vi "Mood Analysis.vi"(2 "Rhythm":dbl[][](array[numeric]), 3 "Timbre":dbl[][](array[numeric]), 4 "Intensity":dbl[][](array[numeric])) -> (0 "Stress":dbl, 1 "Energy":dbl)   [LabVIEW 2013]
panel:
  out "Mood Group":i16(graph)
  out "Stress":dbl(graph)
  out "Energy":dbl(graph)
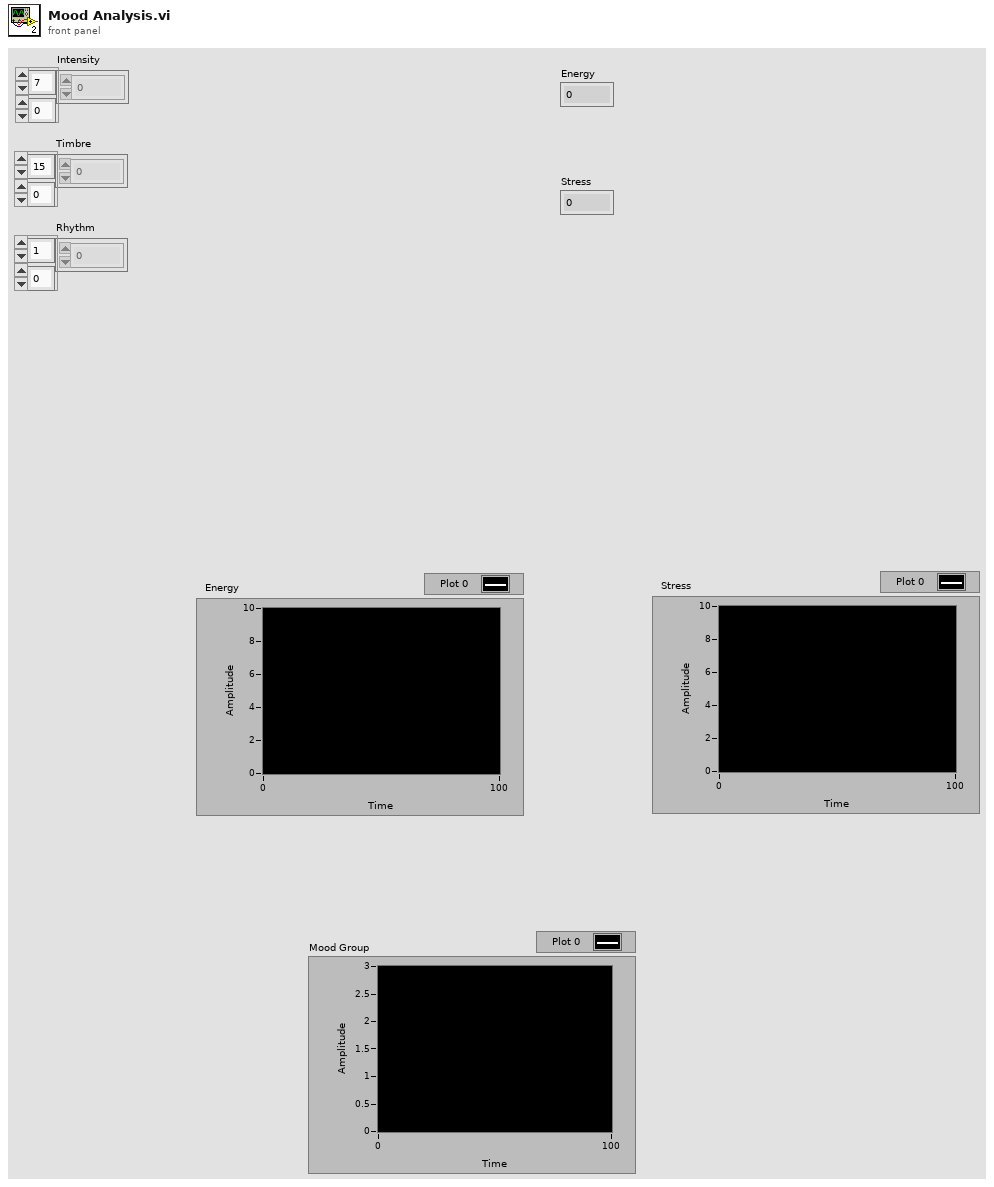
[diagram p1: front panel]
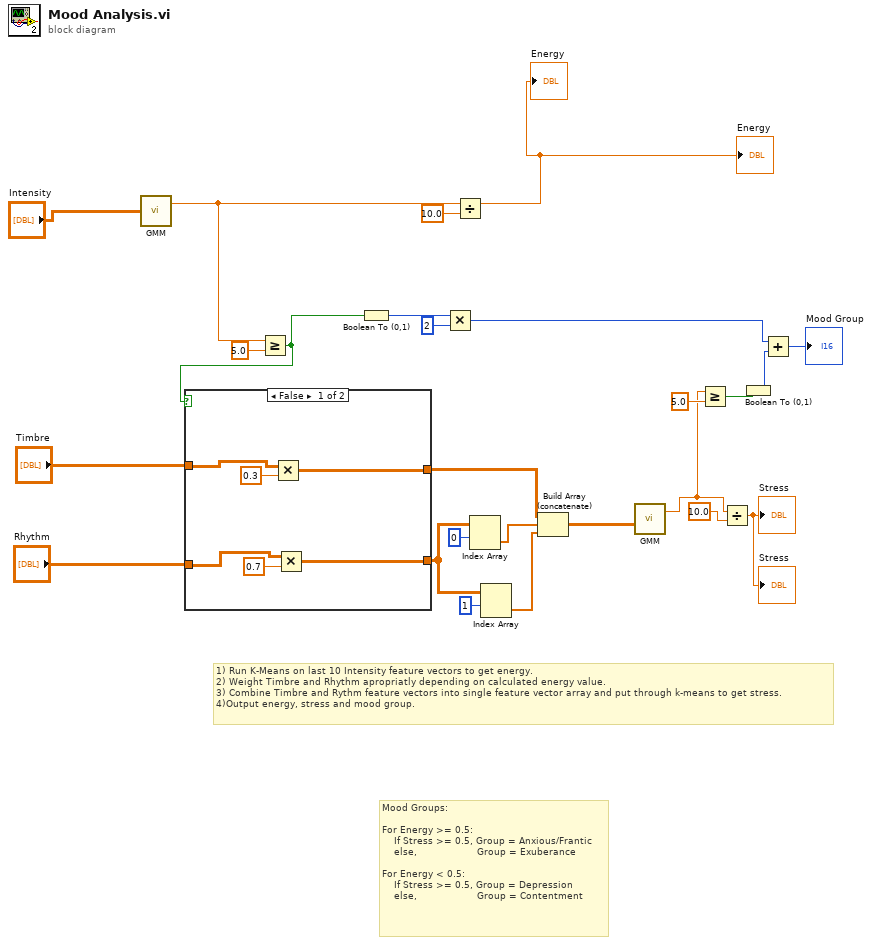
[diagram p0: block diagram]
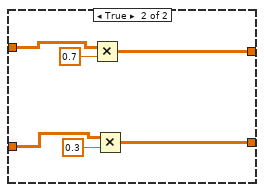
[diagram p2: hidden frame]
diagram:
  # "Mood Groups:\n\nFor Energy >= 0.5:\n    If Stress >= 0.5, Group = Anxious/Frantic\n    else,                    Group = Exuberance\n\nFor Energy < 0.5:\n    If Stress >= 0.5, Group = Depression\n    else,                    Group = Contentment"
  # "1) Run K-Means on last 10 Intensity feature vectors to get energy.\n2) Weight Timbre and Rhythm apropriatly depending on calculated energy value.\n3) Combine Timbre and Rythm feature vectors into single feature vector array and put through k-means to get stress.\n4)Output energy, stress and mood group."
  n1 = call "GMM.vi"("Array"="Intensity") -> ("Group 1"=w14:dbl)  [unwired: 1 out]
  n2 = Greater Or Equal?(x=w14, y=5.0) -> (x >= y?=w12:bool)
  n3 = case shown="False" w12 {
    tunnel: "Timbre" -> [w26 w35]
    tunnel: "Rhythm" -> [w27 w34]
    tunnel: [w29 w33] -> w21
    tunnel: [w28 w32] -> w18
    frame False {
      n4 = Multiply(x=w26, y=0.3) -> (x*y=w29:dbl[][])
      n5 = Multiply(x=w27, y=0.7) -> (x*y=w28:dbl[][])
    }
    frame True {
      n6 = Multiply(x=w35, y=0.7) -> (x*y=w33:dbl[][])
      n7 = Multiply(x=w34, y=0.3) -> (x*y=w32:dbl[][])
    }
  }
  n8 = Boolean To (0,1)(Boolean=w12) -> (0, 1=w11:i16)
  n9 = Multiply(x=w11, y=i16 2) -> (x*y=w9:i16)
  n10 = Divide(x=w14, y=10.0) -> (x/y=→"Energy" →"Energy":dbl)
  n11 = Index Array(array=w18, index (row)=0) -> (element=w16:dbl[])  [unwired: 1 in]
  n12 = Index Array(array=w18, index (row)=1) -> (element=w15:dbl[])  [unwired: 1 in]
  n13 = Build Array (concatenate)(w21, w16, w15) -> (w20:dbl[][])
  n14 = call "GMM.vi"("Array"=w20) -> ("Group 1"=w4:dbl)  [unwired: 1 out]
  n15 = Greater Or Equal?(x=w4, y=5.0) -> (x >= y?=w8:bool)
  n16 = Divide(x=w4, y=10.0) -> (x/y=→"Stress" →"Stress":dbl)
  n17 = Boolean To (0,1)(Boolean=w8) -> (0, 1=w7:i16)
  n18 = Add(x=w9, y=w7) -> (x+y=→"Mood Group":i16)
